vi "Deinit.vi"(8 "error in":errorcluster, 11 "UDP in":refnum<class "UDP.lvclass">) -> (0 "error out":errorcluster, 3 "UDP out":refnum<class "UDP.lvclass">)   [LabVIEW 2020, in "Plugin Instrument Driver.lvlib" / "UDP.lvclass"]
doc: "Close the UDP Connection"
uses:
  UDP.lvclass
  Typedefs/Device Details.ctl
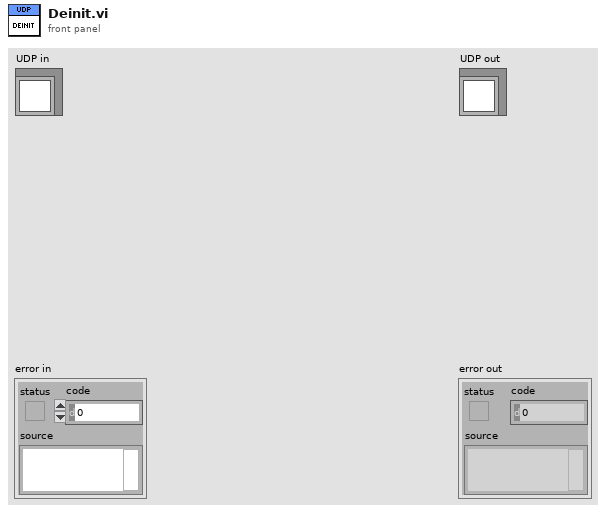
[diagram p1: front panel]
types:
  T1 = typedef "Plugin Instrument Driver.lvlib/UDP.lvclass/Device Details.ctl" = cluster{"Device Port Number":u16, "Device IP":string, "Timeout":i32, "Port Number":u16, "Connection ID":refnum<k16>}
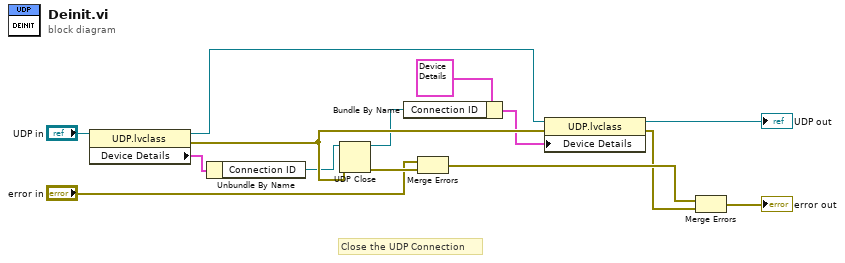
[diagram p0: block diagram]
diagram:
  # "Close the UDP Connection"
  n1 = property class="UDP.lvclass"(reference="UDP in") -> (reference out=w11:refnum<class "UDP.lvclass">, error out=w10:errorcluster, "Device Details"=w5:T1)  [unwired: 1 in]
  n2 = Unbundle By Name(w5) -> ("Connection ID"=w4:refnum<k16>)
  n3 = UDP Close(connection ID=w4, 8:w10) -> (connection ID out=w2:refnum<k16>, error out=w13:errorcluster)
  n4 = Bundle By Name(cluster=T1 {"Device Port Number"=2001, "Device IP"="192.168.1.1.100", "Timeout"=5000, "Port Number"=1234, "Connection ID"=refnum} ("Device Details"), "Connection ID"=w2) -> (w1:T1)
  n5 = Merge Errors("error in", w13) -> (w9:errorcluster)
  n6 = property class="UDP.lvclass"(reference=w11, error in=w10, "Device Details"=w1) -> (reference out=→"UDP out":refnum<class "UDP.lvclass">, error out=w8:errorcluster)
  n7 = Merge Errors(w9, w8) -> (→"error out":errorcluster)
